vi "List VIs without Test Coverage.vi"(8 "error in (no error)":errorcluster, 9 "Tests Root":path, 10 "Source Root":path) -> (0 "error out":errorcluster, 1 "Test VIs":path[](array[path]), 2 "VIs without test coverage":string[](array[string]))   [LabVIEW 2009]
uses:
  <userlib>/_OpenG.lib/array/array.llb/Conditional Auto-Indexing Tunnel (String)__ogtk.vi
  <userlib>/_OpenG.lib/file/file.llb/Build Path - File Names Array__ogtk.vi
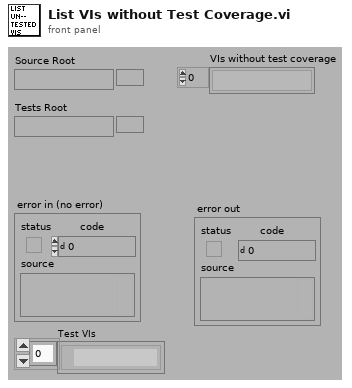
[diagram p1: front panel]
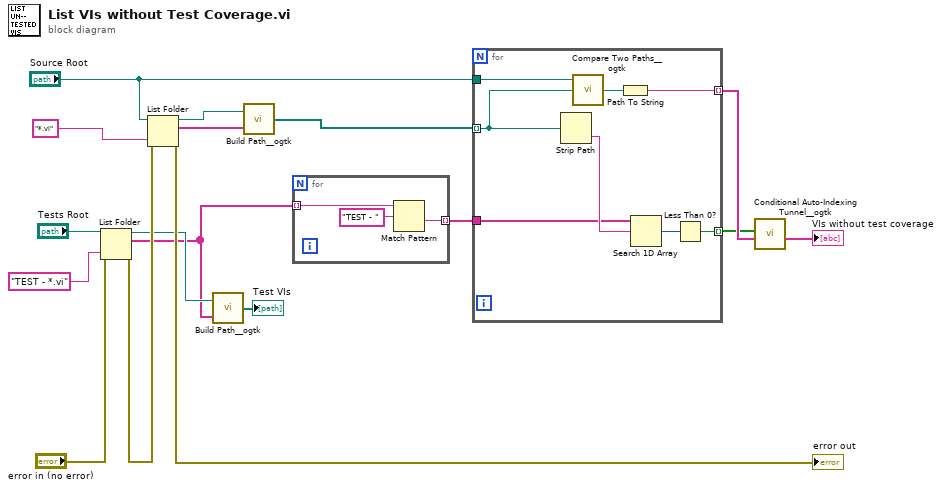
[diagram p0: block diagram]
diagram:
  n1 = List Folder(path="Tests Root", pattern="TEST - *.vi", error in="error in (no error)") -> (path out=w5:path, filenames=w4:string[], error out=w11:errorcluster)  [unwired: 1 in, 1 out]
  n2 = List Folder(path="Source Root", pattern="*.vi", error in=w11) -> (path out=w9:path, filenames=w7:string[], error out=→"error out":errorcluster)  [unwired: 1 in, 1 out]
  n3 = call-poly <userlib>:"Build Path__ogtk.vi"("name or relative path"=w4, "base path"=w5) -> ("appended path"=→"Test VIs":path[])
  n4 = call-poly <userlib>:"Build Path__ogtk.vi"("name or relative path"=w7, "base path"=w9) -> ("appended path"=w8:path[])
  n5 = for {
    tunnel: w4 -> [w20] mode=indexing
    tunnel: [w18] -> w10 mode=indexing
    n6 = Match Pattern(string=w20, regular expression="TEST - ") -> (after substring=w18:string)  [unwired: 1 in, 3 out]
  }
  n7 = for {
    tunnel: w8 -> [w23] mode=indexing
    tunnel: w10 -> [w27]
    tunnel: [w25] -> w15 mode=indexing
    tunnel: "Source Root" -> [w24]
    tunnel: [w21] -> w16 mode=indexing
    n8 = Strip Path(path=w23) -> (name=w28:string)  [unwired: 1 out]
    n9 = call <userlib>:"Compare Two Paths__ogtk.vi"("path2"=w23, "path1"=w24) -> ("relative path from 1 to 2"=w22:path)  [unwired: 1 in, 2 out]
    n10 = Path To String(path=w22) -> (string=w21:string)
    n11 = Search 1D Array(1D array=w27, element=w28) -> (index of element=w26:i32)  [unwired: 1 in]
    n12 = Less Than 0?(x=w26) -> (x < 0?=w25:bool)
  }
  n13 = call-poly <userlib>:"Conditional Auto-Indexing Tunnel__ogtk.vi"("Array in"=w16, "Elements to keep"=w15) -> ("Filtered Array out"=→"VIs without test coverage":string[])  [unwired: 5 in]
